vi "UpdateDeviceImages_1_0.vi"() -> ()   [LabVIEW 2016]
doc: "This is an example of how to read Data Sets from the NI InsightCM database. Using a similiar method you can read any waveform that has been stored and perform additional analysis on it or save it to a file format."
uses:
  <vilib>/addons/InsightCM/MessageBus/MessageService/IcmMessageService.lvclass
  <vilib>/addons/InsightCM/MessageBus/MessageLibrary/SysCfgDeployer/controls/SysCfgDeployPackageRequestBody.ctl
  subVIs/States.ctl
panel:
  in  "stop 2":bool
  in  "stop":bool
  in  "User":string="admin"
  out "Devices To Update - all info":T1[](array[typedef])
  out "Images":string
  out "Current Iteration":i32
  out "Status":string
  out "Total Devices":i32
  out "All Devices":string[](array[string])
  out "Online Devices to Update":i32
  out "BatchDevicesToUpdate":T1[](array[typedef])
  out "SubsetForBatchDeploy":T1[](array[typedef])
  out "SysCfgDeployPackageRequest":T1
  out "error out":errorcluster
  in  "DeployImage":bool
  out "Devices To Update":string[](array[string])
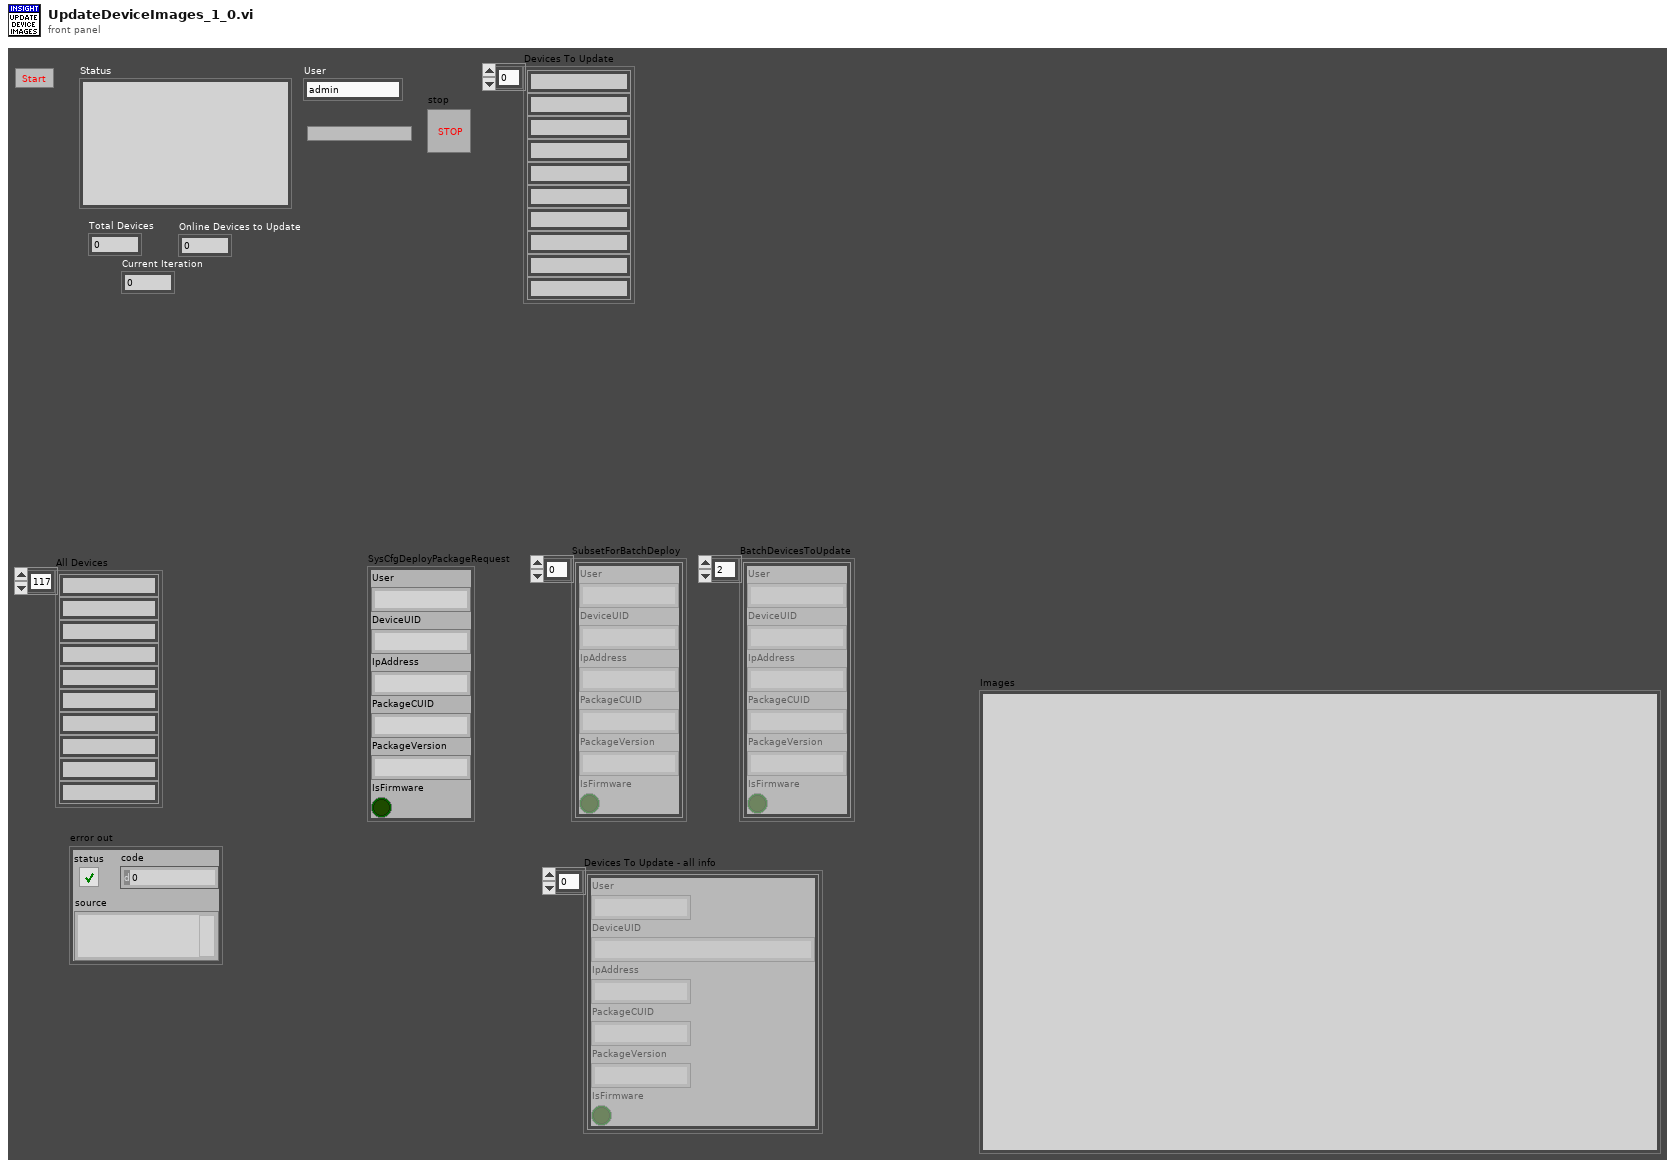
[diagram p1: front panel]
types:
  T1 = typedef "SysCfgDeployPackageRequestBody.ctl" = cluster{"User":string, "DeviceUID":string, "IpAddress":string, "PackageCUID":string, "PackageVersion":string, "IsFirmware":bool}
  T2 = typedef "States.ctl" = enum16{"Deploy", "Wait", "CheckForOnlineDevices", "Init", "DeviceSubset", "ResetSMS", "Check", "Report", "Reset", "ResetConn"}
  T3 = enum8{"Enabled", "Disabled", "Disabled and Grayed Out"}
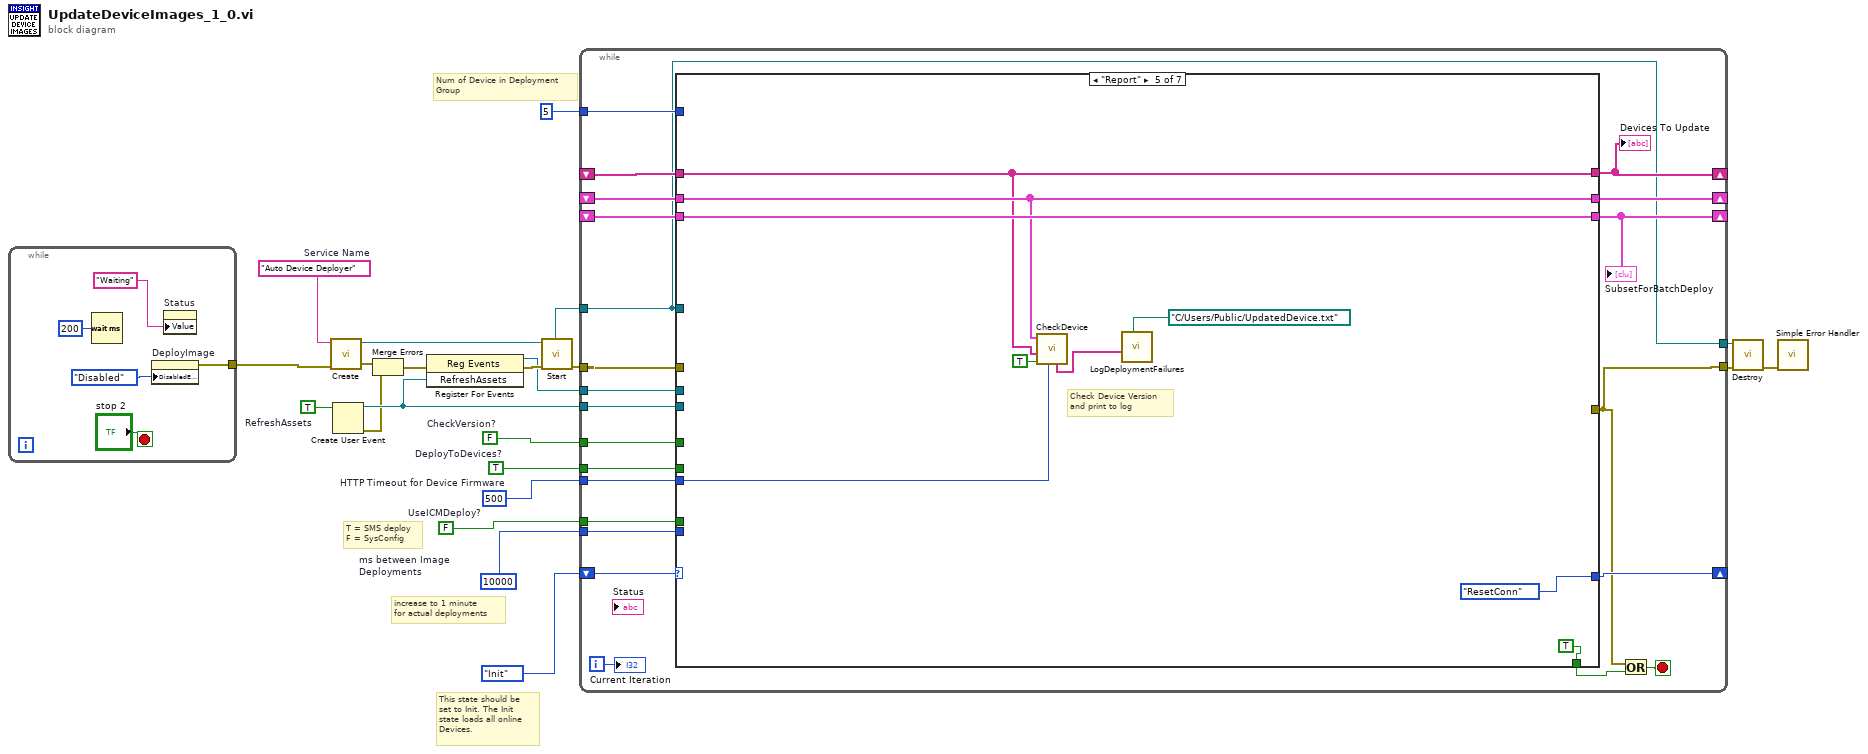
[diagram p0: block diagram]
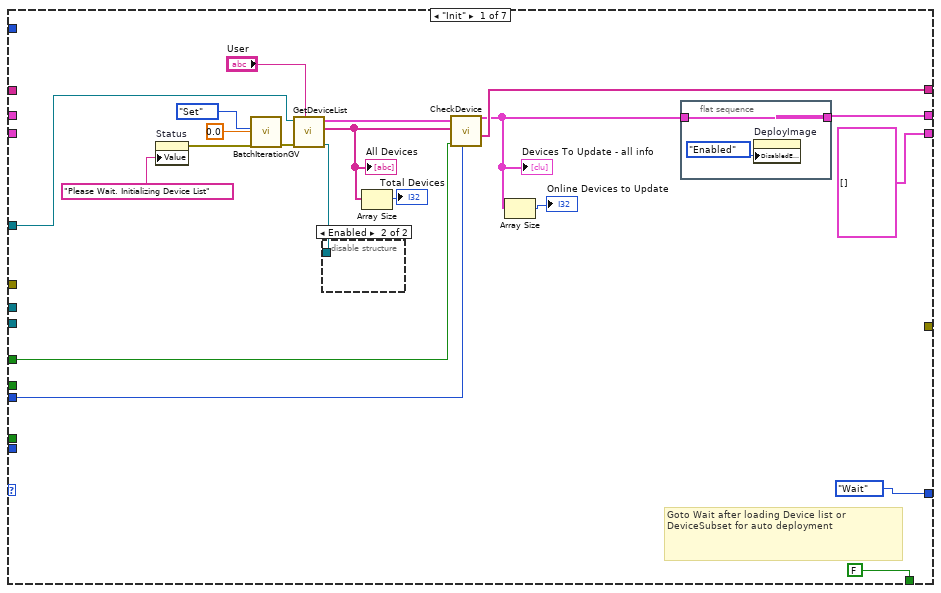
[diagram p2: hidden frame]
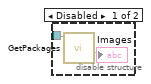
[diagram p3: hidden frame]
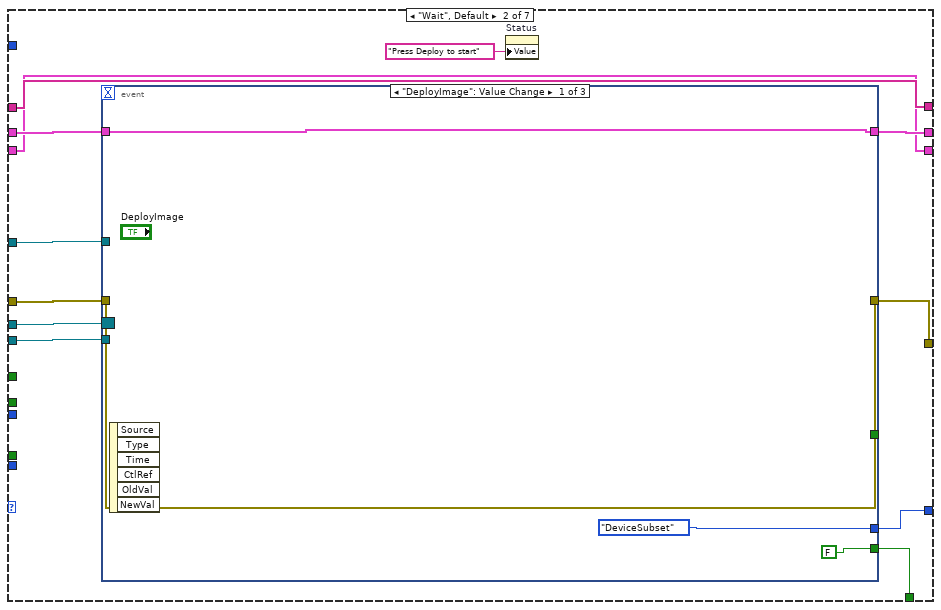
[diagram p4: hidden frame]
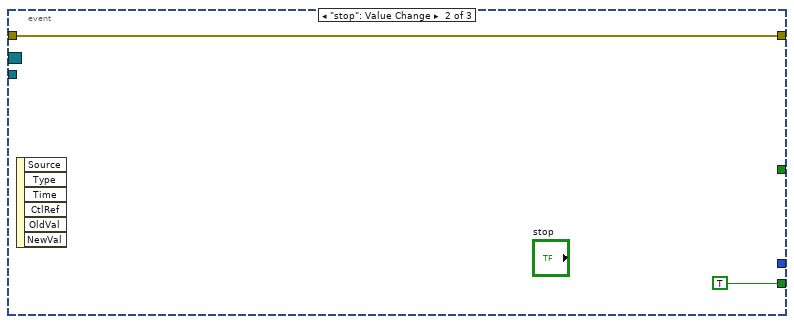
[diagram p5: hidden frame]
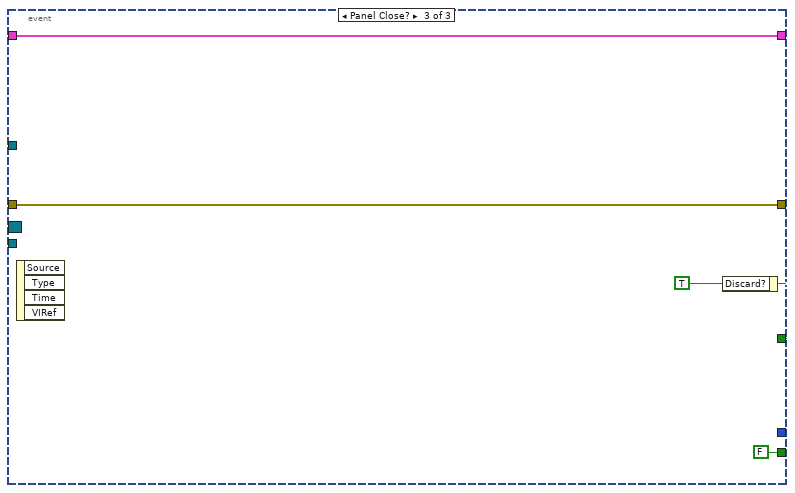
[diagram p6: hidden frame]
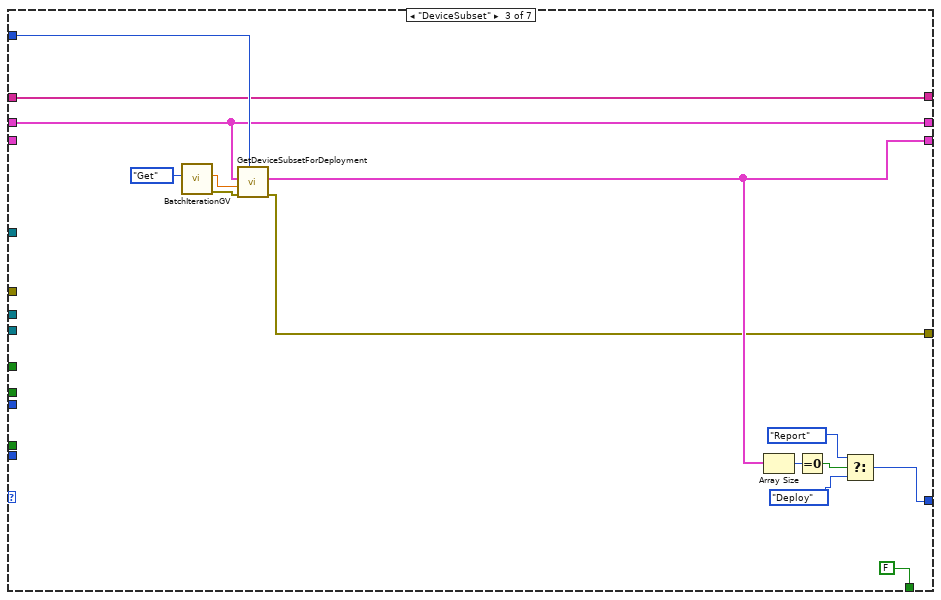
[diagram p7: hidden frame]
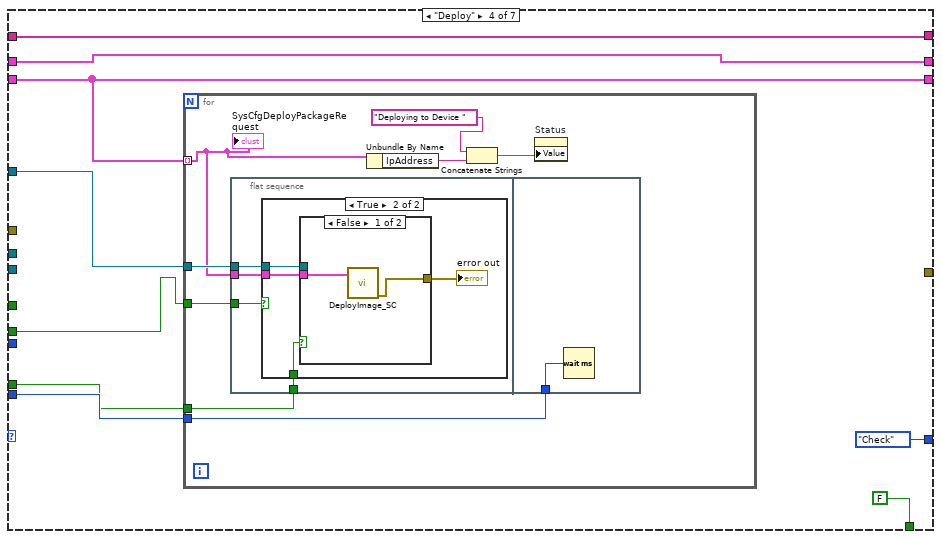
[diagram p8: hidden frame]
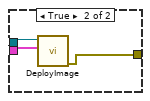
[diagram p10: hidden frame]
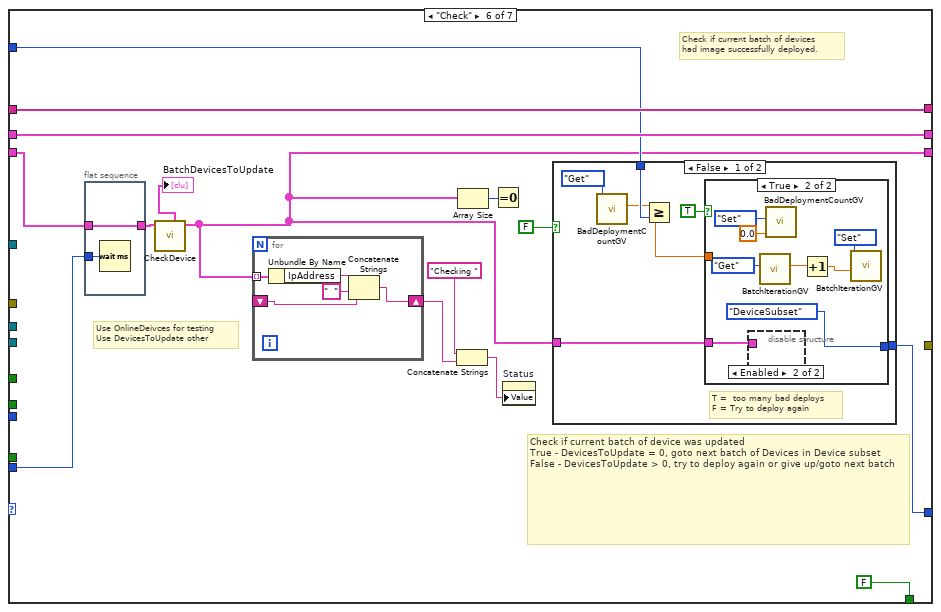
[diagram p11: hidden frame]
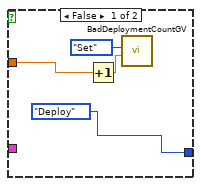
[diagram p12: hidden frame]
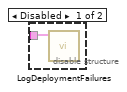
[diagram p13: hidden frame]
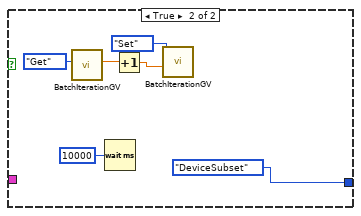
[diagram p14: hidden frame]
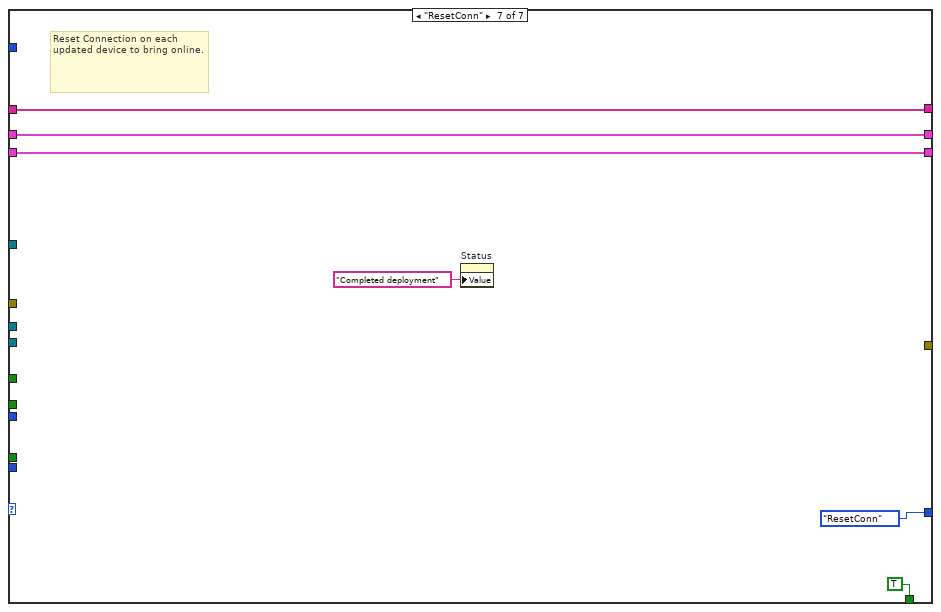
[diagram p15: hidden frame]
diagram:
  w2 = FALSE  # UseICMDeploy?
  w3 = TRUE  # DeployToDevices?
  w4 = FALSE  # CheckVersion?
  w8 = 500  # HTTP Timeout for Device Firmware
  w10 = u32 10000  # ms between Image Deployments
  w19 = TRUE  # RefreshAssets
  w22 = "Auto Device Deployer"  # Service Name
  # "increase to 1 minute\nfor actual deployments"
  # "T = SMS deploy\nF = SysConfig"
  # "This state should be \nset to Init. The Init \nstate loads all online\nDevices."
  # "Num of Device in Deployment\nGroup"
  n1 = while {
    tunnel: [w26] -> w1
    stop <- "stop 2" stop-if-true
    n2 = Wait (ms)(milliseconds to wait=u32 200) -> ()  [unwired: 1 out]
    n3 = property on="DeployImage" class="Bool"("DisabledEnum"=T3."Disabled" ("Disabled")) -> (error out=w26:errorcluster)  [unwired: 2 in, 1 out]
    n4 = property on="Status" class="Str"("Value"="Waiting" ("Status")) -> ()  [unwired: 2 in, 2 out]
  }
  n5 = call <vilib>:"Create.vi"("error in (no error)"=w1, "service name"=w22) -> ("error out"=w15:errorcluster, "service out"=w21:refnum<class "IcmMessageService.lvclass">)  [unwired: 8 in]
  n6 = Create User Event(user event datatype=w19) -> (user event=w16:refnum<user-event>, error out=w14:errorcluster)  [unwired: 1 in]
  n7 = Merge Errors(w15, w14) -> (w13:errorcluster)
  n8 = register-events(error in=w13, w16) -> (reference out=w17:refnum<event-registration>, error out=w18:errorcluster)  [unwired: 1 in]
  n9 = call <vilib>:"Start.vi"("error in (no error)"=w18, "service in"=w21) -> ("error out"=w20:errorcluster, "service out"=w12:refnum<class "IcmMessageService.lvclass">)  [unwired: 8 in]
  n10 = while {
    tunnel: w12 -> [w34]
    tunnel: w20 -> [w49]
    tunnel: w17 -> [w48]
    tunnel: w16 -> [w47]
    shift-right: [w45] -> _
    shift-left: _ -> [w46]
    shift-right: [w43] -> _
    shift-left: States."Init" -> [w44]
    shift-right: [w42] -> _
    shift-left: _ -> [w41]
    shift-right: [w40] -> _
    shift-left: _ -> [w39]
    tunnel: 5 ("num") -> [w38]
    tunnel: w10 -> [w37]
    tunnel: [w29] -> w7
    tunnel: w8 -> [w35]
    tunnel: [w34] -> w5
    tunnel: w4 -> [w33]
    tunnel: w3 -> [w32]
    tunnel: w2 -> [w31]
    i -> [w36]
    stop <- w30 stop-if-true
    n11 = case shown="\"Report\"" w44 {
      tunnel: w49 -> [_ w85 _ _ _ _ _]
      tunnel: [_ w84 w99 _ _ _ _] -> w29
      tunnel: w48 -> [_ w83 _ _ _ _ _]
      tunnel: w47 -> [_ w82 _ _ _ _ _]
      tunnel: w46 -> [_ w81 w98 w117 w147 w163 w201]
      tunnel: w34 -> [w69 w80 _ w118 _ _ _]
      tunnel: [w54 w79 w98 w117 w147 w163 w201] -> w45
      tunnel: [States."Wait" w78 w102 States."Check" States."ResetConn" w160 States."ResetConn"] -> w43
      tunnel: [w65 w77 w108 w116 w145 w164 w200] -> w42
      tunnel: w41 -> [_ w77 w108 w116 w145 w164 w200]
      tunnel: [T1[] [] ("subarray") w76 w103 w115 w149 w154 w202] -> w40
      tunnel: w39 -> [_ w76 _ w115 w149 w157 w202]
      tunnel: w38 -> [_ _ w109 _ _ w161 _]
      tunnel: w37 -> [_ _ _ w114 _ w155 _]
      tunnel: w35 -> [w62 _ _ _ w144 _ _]
      tunnel: w33 -> [w59 _ _ _ _ _ _]
      tunnel: w32 -> [_ _ _ w112 _ _ _]
      tunnel: w31 -> [_ _ _ w111 _ _ _]
      tunnel: [FALSE w74 FALSE FALSE TRUE ("Discard?") FALSE TRUE] -> w28
      frame "Init" {
        # "Goto Wait after loading Device list or\nDeviceSubset for auto deployment"
        n12 = property on="Status" class="Str"("Value"="Please Wait. Initializing Device List" ("Message")) -> (error out=w55:errorcluster)  [unwired: 2 in, 1 out]
        n13 = call "BatchIterationGV.vi"("error in (no error)"=w55, "SetIteration"=0.0, "GetOrSet"=enum16{"Get", "Set"}."Set") -> ("error out"=w56:errorcluster)  [unwired: 6 in, 2 out]
        n14 = call "GetDeviceList.vi"("User"="User", "error in (no error)"=w56, "IcmMessageService in"=w69) -> ("IcmMessageService in 2"=w68:refnum<class "IcmMessageService.lvclass">, "DeviceNames"=w51:string[], "DeviceList"=w63:T1[])  [unwired: 6 in]
        "All Devices" <- w51
        n15 = disable-structure shown="Enabled" {
          disable-tunnel: w68 -> [w71 _]
          frame Disabled {
            n16 = call "GetPackages.vi"("IcmMessageService in"=w71) -> ("string"=→"Images":string)  [unwired: 9 in, 1 out]
          }
          frame Enabled {
          }
        }
        n17 = Array Size(array=w51) -> (size(s)=→"Total Devices":i32)
        n18 = call "CheckDevice.vi"("timeout (10000)"=w62, "CheckVersion"=w59, "DevicesNames"=w51, "DeviceList"=w63) -> ("DevicesToUpdateNames"=w65:string[], "DevicesToUpdate"=w53:T1[])  [unwired: 2 in, 4 out]
        "Devices To Update - all info" <- w53
        n19 = Array Size(array=w53) -> (size(s)=→"Online Devices to Update":i32)
        n20 = flat-sequence {
          tunnel: [w73] -> w54
          tunnel: w53 -> [w73]
          frame #0 {
            n21 = property on="DeployImage" class="Bool"("DisabledEnum"=T3."Enabled" ("Disabled")) -> ()  [unwired: 2 in, 2 out]
          }
        }
      }
      frame "Wait", Default {
        n22 = event shown="[0] \"DeployImage\": Value Change" {
          selector: w83 -> [_ _ _]
          dyn-events: _ -> [_ _ _]
          timeout: _ -> [_ _ _]
          tunnel: w85 -> [w89 w91 w94]
          tunnel: w80 -> [_ _ _]
          tunnel: [_ _ w95] -> _
          tunnel: [w89 w91 w94] -> w84
          tunnel: w82 -> [_ _ _]
          tunnel: w81 -> [w88 _ w93]
          tunnel: [w88 _ w93] -> w79
          tunnel: [States."DeviceSubset" _ _] -> w78
          tunnel: [FALSE TRUE FALSE] -> w74
          event "DeployImage": Value Change {
            n23 = event-data() -> ()  [unwired: 1 in, 6 out]
          }
          event "stop": Value Change {
            n24 = event-data() -> ()  [unwired: 1 in, 6 out]
          }
          event Panel Close? {
            w95 = TRUE ("Discard?")
            n25 = event-data() -> ()  [unwired: 1 in, 4 out]
            n26 = event-data("Discard?"=w95) -> ()  [unwired: 1 in, 1 out]
          }
        }
        n27 = property on="Status" class="Str"("Value"="Press Deploy to start" ("Message")) -> ()  [unwired: 2 in, 2 out]
      }
      frame "DeviceSubset" {
        n28 = call "BatchIterationGV.vi"("GetOrSet"=enum16{"Get", "Set"}."Get") -> ("error out"=w106:errorcluster, "Iteration"=w107:dbl)  [unwired: 8 in, 1 out]
        n29 = call "GetDeviceSubsetForDeployment.vi"("num"=w109, "error in (no error)"=w106, "i"=w107, "DeviceList"=w98) -> ("Error Out"=w99:errorcluster, "subarray"=w103:T1[])  [unwired: 6 in]
        n30 = Array Size(array=w103) -> (size(s)=w104:i32)
        n31 = Equal To 0?(x=w104) -> (x = 0?=w97:bool)
        n32 = Select(t=States."Report", s=w97, f=States."Deploy") -> (s? t:f=w102:T2)
      }
      frame "Deploy" {
        n33 = for {
          tunnel: w118 -> [w126]
          tunnel: w115 -> [w122] mode=indexing
          tunnel: w114 -> [w125]
          tunnel: w112 -> [w124]
          tunnel: w111 -> [w123]
          n34 = flat-sequence {
            tunnel: w122 -> [w130]
            tunnel: w126 -> [w129]
            tunnel: w124 -> [w128]
            tunnel: w123 -> [w127]
            tunnel: w125 -> [w140]
            frame #0 {
              n35 = case shown="True" w128 {
                tunnel: w130 -> [_ w134]
                tunnel: w129 -> [_ w133]
                tunnel: w127 -> [_ w131]
                frame False {
                }
                frame True {
                  n36 = case shown="False" w131 {
                    tunnel: w134 -> [w136 w139]
                    tunnel: w133 -> [_ w138]
                    tunnel: [w135 w137] -> w132
                    frame False {
                      n37 = call "DeployImage_SC.vi"("SysCfgDeployRequest"=w136) -> ("error out"=w135:errorcluster)  [unwired: 10 in]
                    }
                    frame True {
                      n38 = call "DeployImage.vi"("SysCfgDeployPackageRequest"=w139, "service"=w138) -> ("error out"=w137:errorcluster)  [unwired: 9 in]
                    }
                  }
                  "error out" <- w132
                }
              }
            }
            frame #1 {
              n39 = Wait (ms)(milliseconds to wait=w140) -> ()  [unwired: 1 out]
            }
          }
          n40 = Unbundle By Name(w122) -> ("IpAddress"=w121:string)
          n41 = Concatenate Strings("Deploying to Device " ("Message"), w121) -> (w119:string)
          n42 = property on="Status" class="Str"("Value"=w119) -> ()  [unwired: 2 in, 2 out]
          "SysCfgDeployPackageRequest" <- w122
        }
      }
      frame "Report" {
        # "Check Device Version\nand print to log"
        n43 = call "CheckDevice.vi"("timeout (10000)"=w144, "CheckVersion"=TRUE, "DevicesNames"=w145, "DeviceList"=w147) -> ("UpdatedDevicesName"=w146:string[])  [unwired: 2 in, 5 out]
        n44 = call "LogDeploymentFailures.vi"("UpdatedDevices"=path "C:/Users/Public/UpdatedDevice.txt", "Names"=w146) -> ()  [unwired: 10 in]
      }
      frame "Check" {
        # "Use OnlineDeivces for testing\nUse DevicesToUpdate other"
        # "Check if current batch of devices \nhad image successfully deployed."
        # "Check if current batch of device was updated\nTrue - DevicesToUpdate = 0, goto next batch of Devices in Device subset\nFalse - DevicesToUpdate > 0, try to deploy again or give up/goto next batch"
        n45 = flat-sequence {
          tunnel: w157 -> [w171]
          tunnel: [w171] -> w156
          tunnel: w155 -> [w170]
          frame #0 {
            n46 = Wait (ms)(milliseconds to wait=w170) -> ()  [unwired: 1 out]
          }
        }
        n47 = call "CheckDevice.vi"("DeviceList"=w156) -> ("OnlineDevices"=w154:T1[], "DevicesToUpdate"=→"BatchDevicesToUpdate":T1[])  [unwired: 5 in, 4 out]
        n48 = for {
          tunnel: w154 -> [w169] mode=indexing
          shift-right: [w167] -> w153
          shift-left: _ -> [w166]
          n49 = Unbundle By Name(w169) -> ("IpAddress"=w168:string)
          n50 = Concatenate Strings(w168, "  " ("string"), w166) -> (w167:string)
        }
        n51 = Concatenate Strings("Checking " ("Status"), w153) -> (w151:string)
        n52 = Array Size(array=w154) -> (size(s)=w158:i32)
        n53 = Equal To 0?(x=w158) -> ()  [unwired: 1 out]
        n54 = property on="Status" class="Str"("Value"=w151) -> ()  [unwired: 2 in, 2 out]
        n55 = case shown="False" FALSE {
          tunnel: w161 -> [w176 _]
          tunnel: [w174 States."DeviceSubset"] -> w160
          tunnel: w154 -> [w173 _]
          frame False {
            # "T =  too many bad deploys\nF = Try to deploy again"
            n56 = call "BadDeploymentCountGV.vi"("GetOrSet"=enum16{"Get", "Set"}."Get") -> ("BadDeployCount"=w175:dbl)  [unwired: 9 in, 1 out]
            n57 = Greater Or Equal?(x=w175, y=w176) -> ()  [unwired: 1 out]
            n58 = case shown="True" TRUE {
              tunnel: w175 -> [w179 _]
              tunnel: [States."Deploy" States."DeviceSubset"] -> w174
              tunnel: w173 -> [_ w183]
              frame False {
                n59 = Increment(x=w179) -> (x+1=w180:dbl)
                n60 = call "BadDeploymentCountGV.vi"("SetBadDeployments"=w180, "GetOrSet"=enum16{"Get", "Set"}."Set") -> ()  [unwired: 8 in, 2 out]
              }
              frame True {
                n61 = disable-structure shown="Enabled" {
                  disable-tunnel: w183 -> [w190 _]
                  frame Disabled {
                    n62 = call "LogDeploymentFailures.vi"(11:w190) -> ()  [unwired: 11 in]
                  }
                  frame Enabled {
                  }
                }
                n63 = call "BatchIterationGV.vi"("GetOrSet"=enum16{"Get", "Set"}."Get") -> ("Iteration"=w186:dbl)  [unwired: 8 in, 2 out]
                n64 = call "BadDeploymentCountGV.vi"("SetBadDeployments"=0.0, "GetOrSet"=enum16{"Get", "Set"}."Set") -> ()  [unwired: 8 in, 2 out]
                n65 = Increment(x=w186) -> (x+1=w185:dbl)
                n66 = call "BatchIterationGV.vi"("SetIteration"=w185, "GetOrSet"=enum16{"Get", "Set"}."Set") -> ()  [unwired: 7 in, 3 out]
              }
            }
          }
          frame True {
            n67 = call "BatchIterationGV.vi"("GetOrSet"=enum16{"Get", "Set"}."Get") -> ("Iteration"=w195:dbl)  [unwired: 8 in, 2 out]
            n68 = Wait (ms)(milliseconds to wait=u32 10000) -> ()  [unwired: 1 out]
            n69 = Increment(x=w195) -> (x+1=w194:dbl)
            n70 = call "BatchIterationGV.vi"("SetIteration"=w194, "GetOrSet"=enum16{"Get", "Set"}."Set") -> ()  [unwired: 7 in, 3 out]
          }
        }
      }
      frame "ResetConn" {
        # "Reset Connection on each updated device to bring online."
        n71 = property on="Status" class="Str"("Value"="Completed deployment" ("Status")) -> ()  [unwired: 2 in, 2 out]
      }
    }
    "Devices To Update" <- w42
    "SubsetForBatchDeploy" <- w40
    n72 = Or(x=w29, y=w28) -> (x .or. y?=w30:bool)
    "Current Iteration" <- w36
  }
  n73 = call <vilib>:"Destroy.vi"("error in (no error)"=w7, "service in"=w5) -> ("error out"=w6:errorcluster)  [unwired: 9 in]
  n74 = call <vilib>:"Simple Error Handler.vi"("error in (no error)"=w6) -> ()  [unwired: 4 in, 5 out]
